vi "UDP Buffered Tx Process.vi"(10 "Parameters":variant, 11 "Process":refnum<class "Process.lvclass">) -> ()   [LabVIEW 2019, in "UDP-Custom-Device Engine.lvlib"]
uses:
  UDP-Custom-Device Engine.lvlib
  <vilib>/NI/NIVS Inline Async API/_VS Inline Async API/Process/Process.lvclass
  <vilib>/NI/NIVS Inline Async API/_VS Inline Async API/Process/Process.lvclass/Process.ctl
  <vilib>/NI/NIVS Inline Async API/_VS Inline Async API/Process/Data Member Access/Read Data Access.vi
  <vilib>/NI/NIVS Inline Async API/_VS Inline Async API/Error Handling Process/SubVIs/Error.ConvertArray.vi
  <vilib>/NI/NIVS Inline Async API/_Data Access Engine/Data Access Engine/Data Access Engine.lvclass
  <vilib>/NI VeriStand/VeriStand Data/VeriStand Data.lvlib
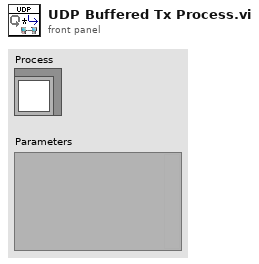
[diagram p1: front panel]
types:
  T1 = typedef "UDP-Custom-Device Engine.lvlib/Engine - Buffered Tx Loop Data.ctl" = cluster{"General Resources":T2, "Header Details":T4, "Buffer Resources":T6, "Runtime Resources":T8, "Echo Resources":T12, "Buffer Option Support":T14, "Channel Resources":T17, "Debug Resources":T20}
  T2 = typedef "UDP-Custom-Device Engine.lvlib/Engine - General Resources.ctl" = cluster{"Packet Name":string, "Packet ID":i32, "Local IP Address":string, "Local Port":i32, "Multicast":bool, "Multicast IP Address":u32, "Header Info":bool[], "Byte Order":enum16{"big-endian, network order", "native, host order", "little-endian"}, "Channel Data Types":T3[], "Duplex Packets":refnum<data-value>}
  T3 = typedef "VeriStand Data.lvlib/Typedefs.Data Types.ctl" = enum16{"Boolean", "Single", "Double", "I8", "I16", "I32", "I64", "U8", "U16", "U32", "U64"}
  T4 = typedef "UDP-Custom-Device Shared.lvlib/Shared - Header Details.ctl" = cluster{"Packet Size":u16, "Protocol Revision":u8, "System Definition Version":u64, "Source Node Name":string, "Packet ID":u32, "Number of Channels":u32, "Static Header Size":u16, "Total Header Size":u16, "CustomHeaderLogic":T5}
  T5 = typedef "UDP-Custom-Device Shared.lvlib/Shared - Custom Header.ctl" = cluster{"CustomHeaderON":bool, "CustomHeaderLogic":string}
  T6 = typedef "UDP-Custom-Device Engine.lvlib/Engine - Buffer Resources.ctl" = cluster{"Data Buffer":u64, "Pointer Encoding":T7, "Buffer Size":u64, "Buffer Size (I32)":i32, "Raw Buffer Data":u8[], "Is Buffered":bool, "External Buffer":bool, "Prepend Header":bool, "Valid Buffer":bool}
  T7 = typedef "UDP-Custom-Device Shared.lvlib/Shared - Pointer Encoding.ctl" = enum16{"Direct Encoding", "Conversion Encoding"}
  T8 = typedef "UDP-Custom-Device Engine.lvlib/Engine - Tx Runtime Resources.ctl" = cluster{"Connection ID":refnum<k16>, "Transmit Option":T9, "Destination IP Address":u32, "Destination Port":u16, "Multicast IP Address":u32, "TTL":u16, "Multicast":bool, "Port as Channel":bool, "ExecutionConfig":T10}
  T9 = typedef "UDP-Custom-Device Shared.lvlib/Shared - Transmit Flag Options.ctl" = enum16{"Always", "One-Shot", "Toggle"}
  T10 = typedef "UDP-Custom-Device Engine.lvlib/Engine - Execution Config.ctl" = cluster{"Loop Period":i64, "RT Loop Period":i64, "Untimed Period":u32, "Target Processor":i32, "Priority":i32, "Thread Management":T11}
  T11 = typedef "UDP-Custom-Device Shared.lvlib/Shared - Thread Management.ctl" = enum16{"Untimed (Default)", "Timed (High Priority)"}
  T12 = typedef "UDP-Custom-Device Engine.lvlib/Engine - Tx Echo Resources.ctl" = cluster{"Transmit Echo Option":T13, "Packet Count":dbl, "Counter Increment":dbl, "Transmit Values":dbl[]}
  T13 = typedef "UDP-Custom-Device Shared.lvlib/Shared - Transmit Echo Options.ctl" = enum16{"PCL Reset", "Counter", "Mirror"}
  T14 = typedef "UDP-Custom-Device Engine.lvlib/Engine - Buffered Tx Buffer Option Support.ctl" = cluster{"Buffer Option":T15, "Sim Option":T16}
  T15 = typedef "UDP-Custom-Device Shared.lvlib/Shared - Transmit Buffer Options.ctl" = enum16{"Static Buffer", "FIFO Buffer", "FIFO Buffer + Port"}
  T16 = typedef "UDP-Custom-Device Shared.lvlib/Shared - Transmit Sim Options.ctl" = enum16{"No Simulation", "Counter", "Full Buffer", "FIFO Test", "FIFO + Port Test"}
  T17 = typedef "UDP-Custom-Device Engine.lvlib/Engine - Buffered Tx Channel Refs.ctl" = cluster{"Transmit Flag":T18, "Transmit Echo":T19, "Transmit Bytes":T18, "Port Channel":T18, "Buffer (External)":T18, "Buffer (Local)":T19, "Timestamp":T18}
  T18 = typedef "Data Access Engine.lvlib/Data Access Engine.lvclass/Read.DVR.ctl" = refnum<data-value>
  T19 = typedef "Data Access Engine.lvlib/Data Access Engine.lvclass/Write.DVR.ctl" = refnum<data-value>
  T20 = typedef "UDP-Custom-Device Engine.lvlib/Engine - Debug Resources.ctl" = cluster{"Debug Mode":bool, "Debug Log File":refnum<file>, "Packet Name":string}
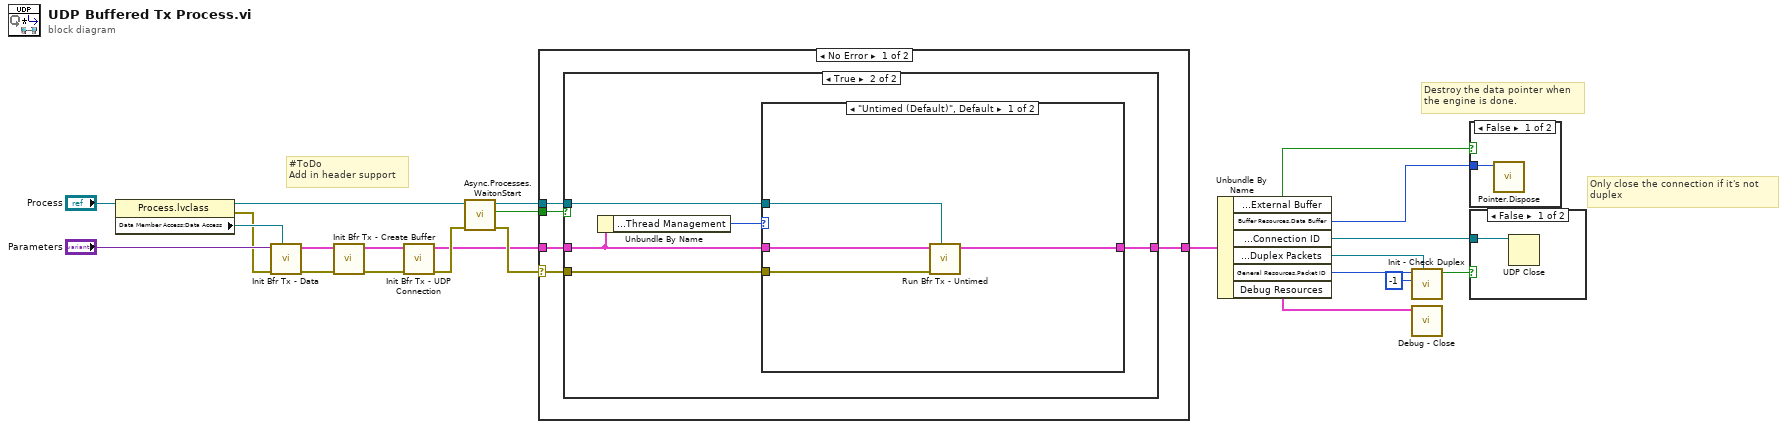
[diagram p0: block diagram]
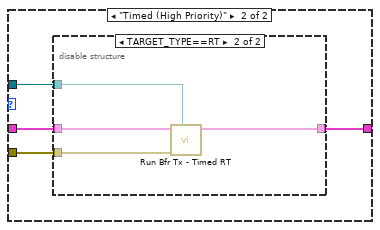
[diagram p3: hidden frame]
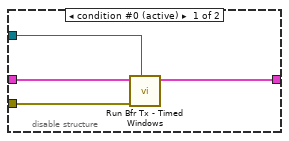
[diagram p4: hidden frame]
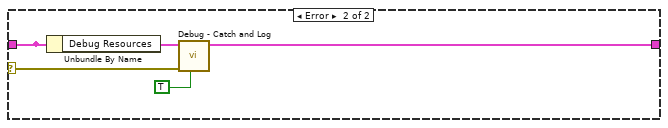
[diagram p5: hidden frame]
diagram:
  # "Only close the connection if it's not\nduplex"
  # "Destroy the data pointer when\nthe engine is done."
  # "#ToDo\nAdd in header support"
  n1 = property class="Process.lvclass"(reference="Process") -> (reference out=w23:refnum<class "Process.lvclass">, error out=w15:errorcluster, "Data Member Access:Data Access"=w16:refnum<class "Data Access Engine.lvclass">)  [unwired: 1 in]
  n2 = call "Init Bfr Tx - Data.vi"("Data Access"=w16, "error in (no error)"=w15, "Parameters"="Parameters") -> ("error out"=w13:errorcluster, "Tx Loop Data"=w14:T1)  [unwired: 7 in]
  n3 = call "Init Bfr Tx - Create Buffer.vi"("error in (no error)"=w13, "Tx Loop Data in"=w14) -> ("error out"=w11:errorcluster, "Tx Loop Data out"=w12:T1)  [unwired: 8 in]
  n4 = call "Init Bfr Tx - UDP Connection.vi"("error in (no error)"=w11, "Tx Loop Data in"=w12) -> ("error out"=w10:errorcluster, "Tx Loop Data out"=w8:T1)  [unwired: 8 in]
  n5 = call <vilib>:"Async.Processes.WaitonStart.vi"("error in (no error)"=w10, "Process"=w23) -> ("error out"=w21:errorcluster, "Execute"=w19:bool, "Process out"=w20:refnum<class "Process.lvclass">)  [unwired: 7 in]
  n6 = case shown="No Error" w21 {
    selector: w21 -> [w26 w53]
    tunnel: w19 -> [w28 _]
    tunnel: w20 -> [w27 _]
    tunnel: w8 -> [w25 w51]
    tunnel: [w24 w51] -> w18
    frame No Error {
      n7 = case shown="True" w28 {
        tunnel: w26 -> [_ w33]
        tunnel: w27 -> [_ w34]
        tunnel: w25 -> [w29 w31]
        tunnel: [w29 w32] -> w24
        frame False {
        }
        frame True {
          n8 = Unbundle By Name(w31) -> ("Runtime Resources.ExecutionConfig.Thread Management"=w30:T11)
          n9 = case shown="\"Untimed (Default)\", Default" w30 {
            tunnel: w34 -> [w36 w42]
            tunnel: w33 -> [w38 w41]
            tunnel: [w35 w40] -> w32
            tunnel: w31 -> [w37 w39]
            frame "Untimed (Default)", Default {
              n10 = call "Run Bfr Tx - Untimed.vi"("Process in"=w36, "error in (no error)"=w38, "Tx Loop Data in"=w37) -> ("Tx Loop Data out"=w35:T1)  [unwired: 8 in]
            }
            frame "Timed (High Priority)" {
              n11 = disable-structure shown="TARGET_TYPE==RT" {
                disable-tunnel: w42 -> [w44 w49]
                disable-tunnel: w41 -> [w45 w48]
                disable-tunnel: w39 -> [w46 w50]
                disable-tunnel: [w43 w47] -> w40
                frame condition #0 (active) {
                  n12 = call "Run Bfr Tx - Timed Windows.vi"("Process in"=w44, "error in (no error)"=w45, "Tx Loop Data in"=w46) -> ("Tx Loop Data out"=w43:T1)  [unwired: 8 in]
                }
                frame condition #1 {
                  n13 = call "Run Bfr Tx - Timed RT.vi"("Process in"=w49, "error in (no error)"=w48, "Tx Loop Data in"=w50) -> ("Tx Loop Data out"=w47:T1)  [unwired: 8 in]
                }
              }
            }
          }
        }
      }
    }
    frame Error {
      n14 = Unbundle By Name(w51) -> ("Debug Resources"=w52:T20)
      n15 = call "Debug - Catch and Log.vi"("Clear Error?"=TRUE, "error in (no error)"=w53, "Debug Resources"=w52) -> ()  [unwired: 8 in, 1 out]
    }
  }
  n16 = Unbundle By Name(w18) -> ("Buffer Resources.External Buffer"=w7:bool, "Buffer Resources.Data Buffer"=w9:u64, "Runtime Resources.Connection ID"=w2:refnum<k16>, "General Resources.Duplex Packets"=w5:refnum<data-value>, "General Resources.Packet ID"=w4:i32, "Debug Resources"=w1:T20)
  n17 = call "Init - Check Duplex.vi"("Duplex Packets"=w5, "Receive Packet ID"=-1, "Transmit Packet ID"=w4) -> ("Is Duplex?"=w3:bool)  [unwired: 6 in, 2 out]
  n18 = call "Debug - Close.vi"("Debug Resources"=w1) -> ()  [unwired: 10 in, 1 out]
  n19 = case shown="False" w7 {
    tunnel: w9 -> [w55 _]
    frame False {
      n20 = call <vilib>:"Pointer.Dispose.vi"("pointer"=w55) -> ()  [unwired: 9 in, 2 out]
    }
    frame True {
    }
  }
  n21 = case shown="False" w3 {
    tunnel: w2 -> [w56 _]
    frame False {
      n22 = UDP Close(connection ID=w56) -> ()  [unwired: 1 in, 2 out]
    }
    frame True {
    }
  }
